vi "Close VI References Set.vi"(8 "error in (no error)":errorcluster, 11 "Engine in":refnum<class "Engine.lvclass">) -> (0 "error out":errorcluster, 3 "Engine out":refnum<class "Engine.lvclass">)   [LabVIEW 2019, in "Engine.lvclass"]
uses:
  Engine.lvclass
  Engine.lvclass/Engine.ctl
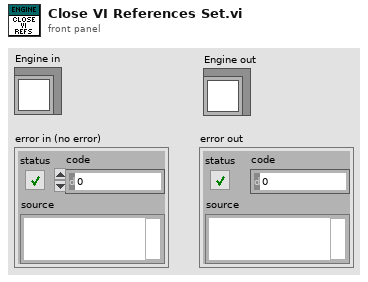
[diagram p1: front panel]
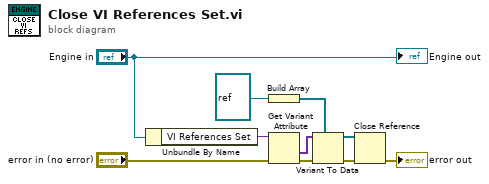
[diagram p0: block diagram]
diagram:
  n1 = Unbundle By Name("Engine in") -> ("VI References Set"=w2:variant)
  n2 = Build Array(refnum<vi> refnum ("This VI")) -> (w5:refnum<vi>[])
  n3 = Get Variant Attribute(Variant=w2, error in="error in (no error)") -> (values=w6:variant[], error out=w8:errorcluster)  [unwired: 2 in, 2 out]
  n4 = Variant To Data(error in=w8, type=w5, Variant=w6) -> (data=w3:refnum<vi>[], error out=w4:errorcluster)
  n5 = Close Reference(reference=w3, error in (no error)=w4) -> (error out=→"error out":errorcluster)
  "Engine out" <- "Engine in"
